vi "HRTF-Read HRTFs.vi"(2 "State":T1, 7 "filestem":string, 11 "error in (no error)":errorcluster) -> (6 "IR":cluster{"offset":dbl, "dx":dbl, "Y":dbl[][]}, 13 "phase":cluster{"offset":dbl, "dx":dbl, "Y":dbl[][]}, 14 "mag":cluster{"offset":dbl, "dx":dbl, "Y":dbl[][]}, 15 "error out":errorcluster)   [LabVIEW 2015]
uses:
  Typedefs/HRTF-State.ctl
  Utility VIs/Math VIs/Linear to dB (scalar).vi
  Utility VIs/Math VIs/FFT x(t) to dB,Degrees (1D).vi
  PXI DAQ VIs/Utility VIs/Array Dimensions (2D).vi
  Utility VIs/Conversion VIs/Create Waveform Cluster (2D).vi
  <vilib>/Analysis/NI_AALPro.lvlib
panel:
  out "error out":errorcluster
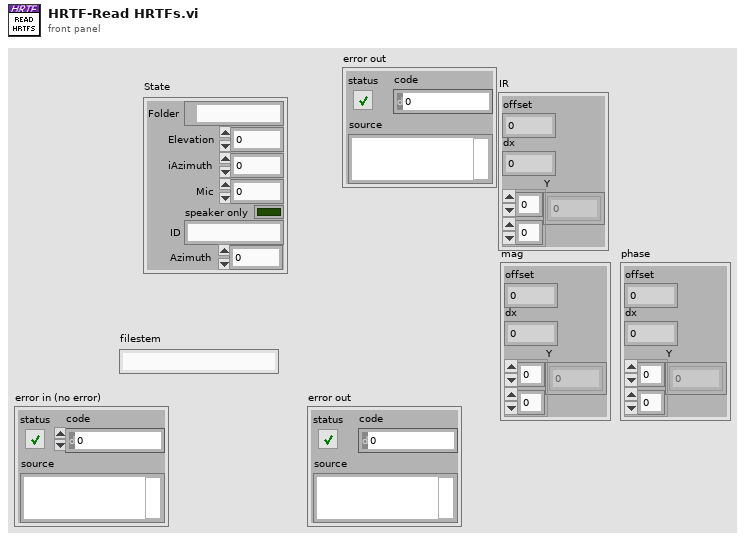
[diagram p1: front panel]
types:
  T1 = typedef "HRTF-State.ctl" = cluster{"Folder":path, "Elevation":dbl, "iAzimuth":i32, "Mic":i32, "speaker only":bool, "ID":string, "Azimuth":dbl}
  T2 = typedef "HRTF-filt Cluster.ctl" = cluster{"Type":string, "Fs":dbl, "a":dbl[], "b":dbl[], "window":i32, "Length_ms":dbl, "Center_ms":dbl}
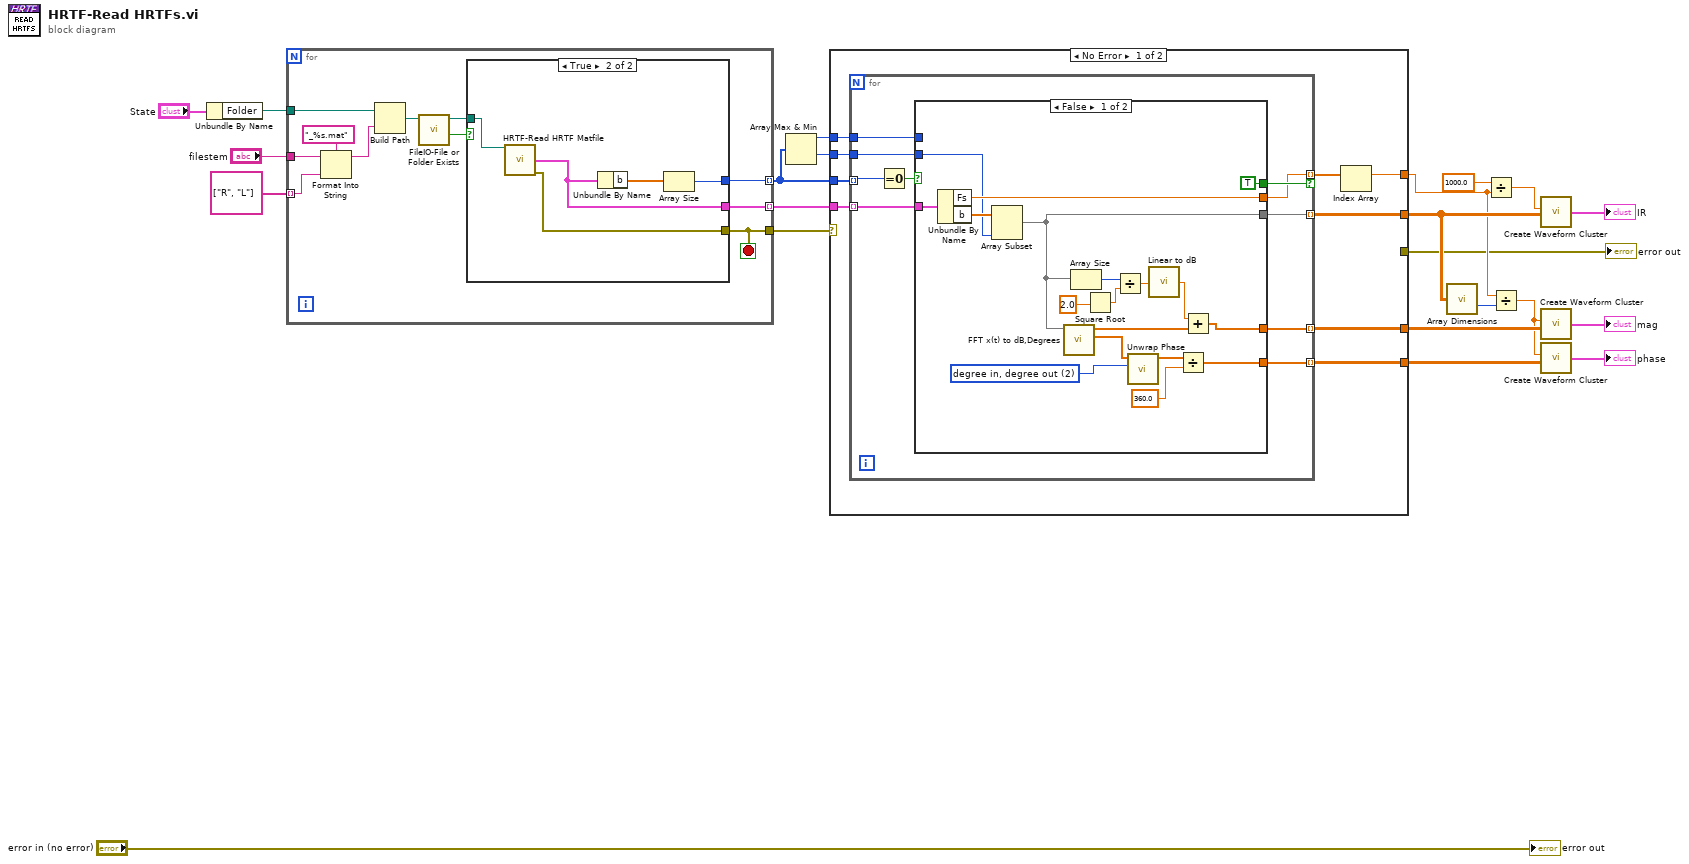
[diagram p0: block diagram]
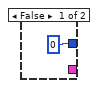
[diagram p2: hidden frame]
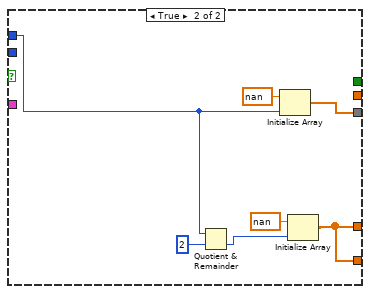
[diagram p3: hidden frame]
diagram:
  n1 = Unbundle By Name("State") -> ("Folder"=w19:path)
  n2 = for {
    tunnel: string[] ["R", "L"] -> [w31] mode=indexing
    tunnel: w19 -> [w30]
    tunnel: "filestem" -> [w33]
    tunnel: [w28] -> w16 mode=indexing
    tunnel: [w23] -> w17
    tunnel: [w24] -> w14 mode=indexing
    stop <- w23 stop-if-true
    n3 = Format Into String(format string="_%s.mat", initial string=w33, w31) -> (resulting string=w29:string)  [unwired: 1 in, 1 out]
    n4 = Build Path(base path=w30, name or relative path=w29) -> (appended path=w27:path)
    n5 = call "FileIO-File or Folder Exists.vi"("path"=w27) -> ("Exists?"=w25:bool, "dup path"=w26:path)  [unwired: 7 in, 2 out]
    n6 = case shown="True" w25 {
      tunnel: w26 -> [_ w39]
      tunnel: [_ w37] -> w28
      tunnel: [_ w38] -> w23
      tunnel: [0 w35] -> w24
      frame False {
      }
      frame True {
        n7 = call "HRTF-Read HRTF Matfile.vi"("path"=w39) -> ("filt"=w37:T2, "error out"=w38:errorcluster)  [unwired: 13 in]
        n8 = Unbundle By Name(w37) -> ("b"=w36:dbl[])
        n9 = Array Size(array=w36) -> (size(s)=w35:i32)
      }
    }
  }
  n10 = Array Max & Min(array=w14) -> (max value=w15:i32, min value=w6:i32)  [unwired: 2 out]
  n11 = case shown="No Error" w17 {
    selector: w17 -> [_ w84]
    tunnel: w16 -> [w48 _]
    tunnel: w15 -> [w47 _]
    tunnel: w14 -> [w46 _]
    tunnel: [_ w84] -> w1
    tunnel: [w45 _] -> w13
    tunnel: [w44 _] -> w12
    tunnel: [w43 _] -> w11
    tunnel: [w41 _] -> w7
    tunnel: w6 -> [w40 _]
    frame No Error {
      n12 = for {
        tunnel: w48 -> [w55] mode=indexing
        tunnel: w47 -> [w57]
        tunnel: w46 -> [w56] mode=indexing
        tunnel: [w54] -> w45 mode=indexing
        tunnel: [w53] -> w44 mode=indexing
        tunnel: [w52] -> w43 mode=indexing
        tunnel: [w50] -> w42 mode=indexing if=w51
        tunnel: w40 -> [w49]
        n13 = Equal To 0?(x=w56) -> (x = 0?=w58:bool)
        n14 = case shown="False" w58 {
          tunnel: w57 -> [_ w79]
          tunnel: w55 -> [w76 _]
          tunnel: [w59 w82] -> w54
          tunnel: [w75 w80] -> w53
          tunnel: [w74 w80] -> w52
          tunnel: [TRUE _] -> w51
          tunnel: [w72 _] -> w50
          tunnel: w49 -> [w60 _]
          frame False {
            w69 = 2 items=["radian in, radian out", "radian in, degree out", "degree in, degree out", "degree in, radian out"] ("phase unit")
            n15 = Unbundle By Name(w76) -> ("Fs"=w72:dbl, "b"=w61:dbl[])
            n16 = Array Subset(array=w61, length=w60) -> (w59:dbl[])  [unwired: 1 in]
            n17 = call-poly "FFT x(t) to dB,Degrees.vi"("X"=w59) -> ("+Freq Phase of FFT (degrees)"=w70:dbl[], "+Freq. Mag of FFT (dB rms)"=w67:dbl[])  [unwired: 8 in, 1 out]
            n18 = Array Size(array=w59) -> (size(s)=w66:i32)
            n19 = Square Root(x=2.0) -> (sqrt(x)=w65:dbl)
            n20 = Divide(x=w66, y=w65) -> (x/y=w63:dbl)
            n21 = call <vilib>:"Unwrap Phase.vi"("phase unit"=w69, "Phase"=w70) -> ("Unwrapped Phase"=w71:dbl[])  [unwired: 8 in, 1 out]
            n22 = call-poly "Linear to dB.vi"("Linear"=w63) -> ("dB"=w62:dbl)
            n23 = Divide(x=w71, y=360.0) -> (x/y=w74:dbl[])
            n24 = Add(x=w62, y=w67) -> (x+y=w75:dbl[])
          }
          frame True {
            n25 = Quotient & Remainder(x=w79, y=2) -> (floor(x/y)=w77:i32)  [unwired: 1 out]
            n26 = Initialize Array(nan, w79) -> (w82:dbl[])
            n27 = Initialize Array(nan, w77) -> (w80:dbl[])
          }
        }
      }
      n28 = Index Array(array=w42) -> (element=w41:dbl)  [unwired: 1 in]
    }
    frame Error {
    }
  }
  "error out" <- w1
  n29 = call-poly "Array Dimensions.vi"("2D Array"=w13) -> ("# columns"=w3:i32)  [unwired: 13 in, 1 out]
  n30 = Divide(x=1000.0, y=w7) -> (x/y=w4:dbl)
  n31 = Divide(x=w7, y=w3) -> (x/y=w2:dbl)
  n32 = call-poly "Create Waveform Cluster.vi"("dx"=w4, "Array"=w13) -> ("waveform cluster"=→"IR":cluster{"offset":dbl, "dx":dbl, "Y":dbl[][]})  [unwired: 3 in]
  n33 = call-poly "Create Waveform Cluster.vi"("dx"=w2, "Array"=w12) -> ("waveform cluster"=→"mag":cluster{"offset":dbl, "dx":dbl, "Y":dbl[][]})  [unwired: 3 in]
  n34 = call-poly "Create Waveform Cluster.vi"("dx"=w2, "Array"=w11) -> ("waveform cluster"=→"phase":cluster{"offset":dbl, "dx":dbl, "Y":dbl[][]})  [unwired: 3 in]
  "error out" <- "error in (no error)"
